vi "Magazine_Execute.vi"() -> ()   [LabVIEW 2019]
uses:
  Magazine_Cluster.ctl
  Magazine_States.ctl
  Utility VIs/Basic_Motor_Modes.ctl
  Globals/Magazine_Globals.vi
  Globals/Flywheel_Globals.vi
panel:
  in  "Magazine_Firing_Throttle":dbl=0.6
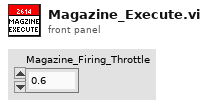
[diagram p1: front panel]
types:
  T1 = typedef "Magazine_Cluster.ctl" = cluster{"Control_States":T2, "Magazine_Throttle":dbl, "Firing":bool}
  T2 = typedef "Magazine_States.ctl" = enum16{"No-Op", "Manual_%Vbus", "Firing", ""}
  T3 = typedef "Basic_Motor_Modes.ctl" = enum16{"Percent_Voltage", "Speed_Control", "Position_Control", "Current"}
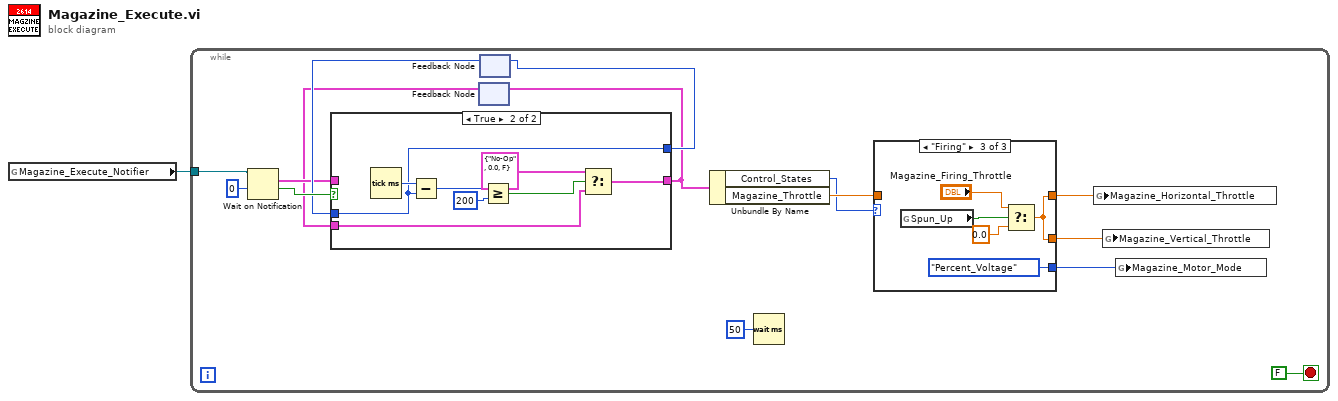
[diagram p0: block diagram]
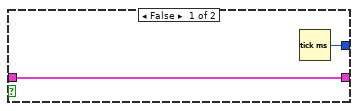
[diagram p2: hidden frame]
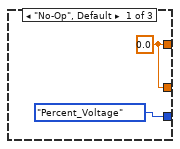
[diagram p3: hidden frame]
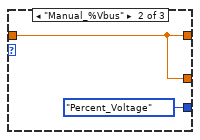
[diagram p4: hidden frame]
diagram:
  n1 = global read "Magazine_Globals.vi" "Magazine_Execute_Notifier"() -> (w1:refnum<notifier>)
  n2 = while {
    tunnel: w1 -> [w4]
    stop <- FALSE stop-if-true
    n3 = Wait on Notification(notifier=w4, timeout in ms (-1)=0) -> (notification=w6:T1, timed out?=w9:bool)  [unwired: 2 in, 2 out]
    n4 = feedback #1() -> (w5:T1)  [unwired: 1 in]
    n5 = feedback #2() -> (w7:u32)  [unwired: 1 in]
    n6 = case shown="True" w9 {
      tunnel: w6 -> [w18 _]
      tunnel: [w18 w26] -> w3
      tunnel: w5 -> [_ w25]
      tunnel: [w17 w23] -> w8
      tunnel: w7 -> [_ w23]
      frame False {
        n7 = Tick Count (ms)() -> (millisecond timer value=w17:u32)
      }
      frame True {
        n8 = Tick Count (ms)() -> (millisecond timer value=w24:u32)
        n9 = Subtract(x=w24, y=w23) -> (x-y=w21:u32)
        n10 = Greater Or Equal?(x=w21, y=u32 200) -> (x >= y?=w22:bool)
        n11 = Select(t=T1 {"Control_States"=enum."No-Op", "Magazine_Throttle"=0.0, "Firing"=FALSE} ("Cluster"), s=w22, f=w25) -> (s? t:f=w26:T1)
      }
    }
    n12 = feedback-in #1(w3) -> ()
    n13 = feedback-in #2(w8) -> ()
    n14 = Unbundle By Name(w3) -> ("Control_States"=w2:T2, "Magazine_Throttle"=w14:dbl)
    n15 = Wait (ms)(milliseconds to wait=u32 50) -> ()  [unwired: 1 out]
    n16 = case shown="\"Firing\"" w2 {
      tunnel: w14 -> [_ w29 _]
      tunnel: [w28 w29 w31] -> w13
      tunnel: [w28 w29 w31] -> w12
      tunnel: [Basic_Motor_Modes."Percent_Voltage" ("Magazine_Motor_Mode") Basic_Motor_Modes."Percent_Voltage" ("Magazine_Motor_Mode") Basic_Motor_Modes."Percent_Voltage" ("Magazine_Motor_Mode")] -> w11
      frame "No-Op", Default {
        w28 = 0.0 ("Magazine_Throttle")
      }
      frame "Manual_%Vbus" {
      }
      frame "Firing" {
        n17 = global read "Flywheel_Globals.vi" "Spun_Up"() -> (w34:bool)
        n18 = Select(t="Magazine_Firing_Throttle", s=w34, f=0.0) -> (s? t:f=w31:dbl)
      }
    }
    n19 = global write "Magazine_Globals.vi" "Magazine_Horizontal_Throttle"(w13) -> ()
    n20 = global write "Magazine_Globals.vi" "Magazine_Vertical_Throttle"(w12) -> ()
    n21 = global write "Magazine_Globals.vi" "Magazine_Motor_Mode"(w11) -> ()
  }
